vi "TablePicture.vi"(4 "RowIndex":i32, 5 "Font In":refnum<class "Font.lvclass">, 6 "Row Configuration":T1={"Cell Defaults"={"Background Color"=16777215, "Horizontal Align"=3, "Vertical Align"=1, "Minimum Height"=0.0, "Fixed Height"=0.0, "Padding"={"Left"=2.0, "Top"=2.0, "Right"=2.0, "Bottom"=3.0}}, "Row Borders"={"Left"={"Enabled"=TRUE, "Width"=0.5, "Color"=0}, "Top"={"Enabled"=TRUE, "Width"=0.75, "Color"=0}, "Right"={"Enabled"=TRUE, "Width"=0.5, "Color"=0}, "Bottom"={"Enabled"=TRUE, "Width"=0.75, "Color"=0}, "Middle Vertical"={"Enabled"=TRUE, "Width"=0.5, "Color"=0}}} {"Cell Defaults"."Vertical Align" items=["Bottom", "Middle", "Top"]; "Cell Defaults"."Horizontal Align" items=["Center", "Justified", "JustifiedAll", "Left", "Right"]}, 7 "TablePictures empty?":bool, 8 "Fehler (Eingang, kein Fehler)":errorcluster, 9 "Table in":string[](array[string]), 10 "TablePictures in":T4={"Ctl Refnum In"=[], "RowOrColumn"=enum."Row", "IndexToInsert"=0, "Image Scale (%)"=[], "Autoscale? (T)"=[], "Horizontal Align"=3} {"Horizontal Align" items=["Center", "Justified", "JustifiedAll", "Left", "Right"]}, 11 "Table Builder (Eingang)":refnum<class "Table Builder.lvclass">) -> (0 "Fehler (Ausgang)":errorcluster, 2 "Row Formatting out":refnum<class "Formatting.lvclass">[](array[class]), 3 "Table Builder (Ausgang)":refnum<class "Table Builder.lvclass">)   [LabVIEW 2020, in "PDF Interface.lvlib" / "PDF Interface Helper.lvlib"]
uses:
  PDF Interface Helper.lvlib
  <vilib>/Simplicity AI/SAI_PDF_API/Classes/Table Formatting/Formatting.lvclass
  <vilib>/Simplicity AI/SAI_PDF_API/Classes/Table Builder/Table Builder.lvclass
  PDFTablePictures.ctl
  <vilib>/Simplicity AI/SAI_PDF_API/Classes/Table Builder/Controls/SAI_PDF_Row Configuration.ctl
  <vilib>/Simplicity AI/SAI_PDF_API/Classes/Table Builder/Controls/SAI_PDF_Default Cell Format.ctl
  <vilib>/Simplicity AI/SAI_PDF_API/Classes/Table Builder/Controls/SAI_PDF_BorderLine.ctl
  <vilib>/Simplicity AI/SAI_PDF_API/Classes/Font/Font.lvclass
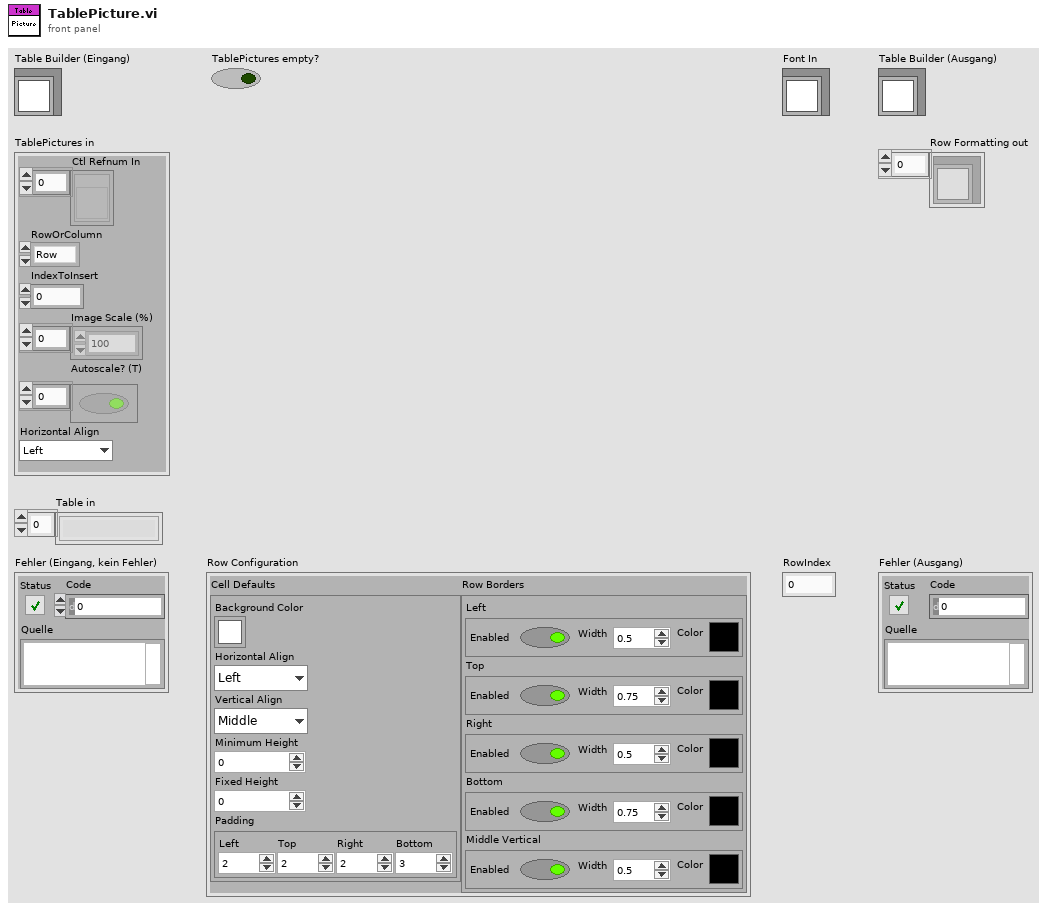
[diagram p1: front panel]
types:
  T1 = typedef "SAI_PDF_Toolkit.lvlib/Table Builder.lvclass/SAI_PDF_Row Configuration.ctl" = cluster{"Cell Defaults":T2, "Row Borders":cluster{"Left":T3, "Top":T3, "Right":T3, "Bottom":T3, "Middle Vertical":T3}}
  T2 = typedef "SAI_PDF_Toolkit.lvlib/Table Builder.lvclass/SAI_PDF_Default Cell Format.ctl" = cluster{"Background Color":u32, "Horizontal Align":i32, "Vertical Align":i32, "Minimum Height":sgl, "Fixed Height":sgl, "Padding":cluster{"Left":sgl, "Top":sgl, "Right":sgl, "Bottom":sgl}}
  T3 = typedef "SAI_PDF_Toolkit.lvlib/Table Builder.lvclass/SAI_PDF_BorderLine.ctl" = cluster{"Enabled":bool, "Width":sgl, "Color":u32}
  T4 = typedef "PDF Interface.lvlib/PDF Interface Helper.lvlib/PDFTablePictures.ctl" = cluster{"Ctl Refnum In":refnum<vi>[], "RowOrColumn":enum16{"Row", "Column"}, "IndexToInsert":u16, "Image Scale (%)":sgl[], "Autoscale? (T)":bool[], "Horizontal Align":i32}
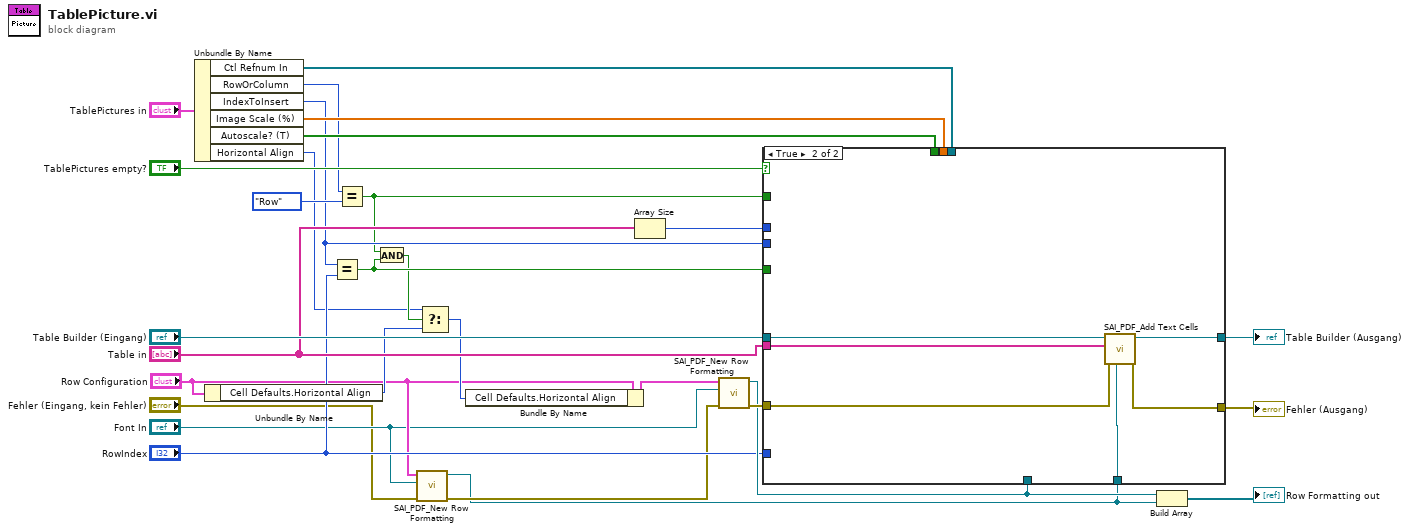
[diagram p0: block diagram]
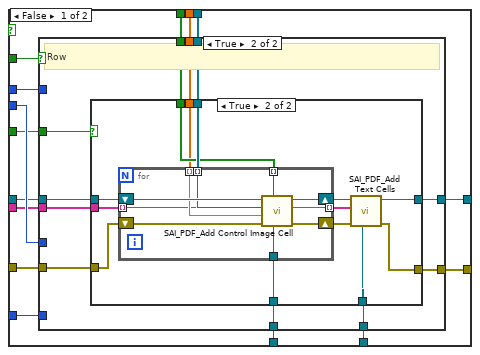
[diagram p2: hidden frame]
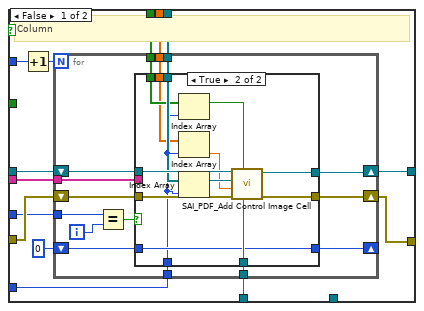
[diagram p3: hidden frame]
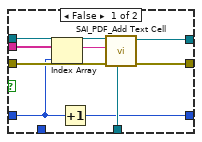
[diagram p4: hidden frame]
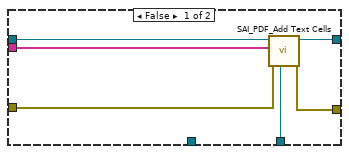
[diagram p5: hidden frame]
diagram:
  n1 = Unbundle By Name("TablePictures in") -> ("Ctl Refnum In"=w24:refnum<vi>[], "RowOrColumn"=w20:enum16{"Row", "Column"}, "IndexToInsert"=w14:u16, "Image Scale (%)"=w23:sgl[], "Autoscale? (T)"=w22:bool[], "Horizontal Align"=w9:i32)
  n2 = Unbundle By Name("Row Configuration") -> ("Cell Defaults.Horizontal Align"=w8:i32)
  n3 = Equal?(x=w14, y="RowIndex") -> (x = y?=w11:bool)
  n4 = Equal?(x=w20, y=enum16{"Row", "Column"}."Row") -> (x = y?=w12:bool)
  n5 = And(x=w12, y=w11) -> (x .and. y?=w10:bool)
  n6 = call <vilib>:"SAI_PDF_New Row Formatting.vi"("error in"="Fehler (Eingang, kein Fehler)", "Font In"="Font In", "Row Configuration"="Row Configuration") -> ("error out"=w3:errorcluster, "Row Formatting"=w1:refnum<class "Formatting.lvclass">)  [unwired: 7 out]
  n7 = Select(t=w9, s=w10, f=w8) -> (s? t:f=w7:i32)
  n8 = Bundle By Name(cluster="Row Configuration", "Cell Defaults.Horizontal Align"=w7) -> (w13:T1)
  n9 = Array Size(array="Table in") -> (size(s)=w18:i32)
  n10 = call <vilib>:"SAI_PDF_New Row Formatting.vi"("error in"=w3, "Font In"="Font In", "Row Configuration"=w13) -> ("error out"=w17:errorcluster, "Row Formatting"=w16:refnum<class "Formatting.lvclass">)  [unwired: 7 out]
  n11 = case shown="True" "TablePictures empty?" {
    tunnel: "Table Builder (Eingang)" -> [w41 w140]
    tunnel: "Table in" -> [w35 w139]
    tunnel: [w39 w138] -> w27
    tunnel: [w37 w137] -> w28
    tunnel: w17 -> [w38 w136]
    tunnel: w1 -> [w36 w135]
    tunnel: w12 -> [w44 _]
    tunnel: "RowIndex" -> [w43 _]
    tunnel: w14 -> [w42 _]
    tunnel: w16 -> [w40 _]
    tunnel: w24 -> [w34 _]
    tunnel: w23 -> [w33 _]
    tunnel: w22 -> [w32 _]
    tunnel: w18 -> [w31 _]
    tunnel: w11 -> [w30 _]
    frame False {
      n12 = case shown="True" w44 {
        tunnel: w43 -> [w50 _]
        tunnel: w42 -> [w52 _]
        tunnel: w41 -> [w57 w106]
        tunnel: w40 -> [w58 w105]
        tunnel: [w56 w104] -> w39
        tunnel: w38 -> [w54 w103]
        tunnel: [w53 w102] -> w37
        tunnel: w36 -> [_ w101]
        tunnel: w35 -> [w55 w100]
        tunnel: w34 -> [w51 w99]
        tunnel: w33 -> [w47 w98]
        tunnel: w32 -> [w48 w97]
        tunnel: w31 -> [w46 _]
        tunnel: w30 -> [_ w96]
        frame False {
          # "Column"
          n13 = Increment(x=w46) -> (x+1=w45:i32)
          n14 = for {
            N: w45 -> [_]
            tunnel: w58 -> [w73]
            shift-right: [w68] -> w56
            shift-left: w57 -> [w72]
            tunnel: w55 -> [w71]
            shift-right: [w69] -> w53
            shift-left: w54 -> [w70]
            tunnel: w52 -> [w66]
            tunnel: w51 -> [w65]
            tunnel: w50 -> [w64]
            shift-right: [w62] -> _
            shift-left: 0 -> [w61]
            tunnel: w48 -> [w60]
            tunnel: w47 -> [w59]
            i -> [w63]
            n15 = Equal?(x=w66, y=w63) -> (x = y?=w67:bool)
            n16 = case shown="True" w67 {
              tunnel: w73 -> [w82 w91]
              tunnel: w72 -> [w81 w95]
              tunnel: w71 -> [w80 _]
              tunnel: w70 -> [w79 w93]
              tunnel: [w78 w92] -> w69
              tunnel: [w77 w94] -> w68
              tunnel: w65 -> [_ w90]
              tunnel: w64 -> [_ w83]
              tunnel: w61 -> [w75 w88]
              tunnel: [w74 w88] -> w62
              tunnel: w60 -> [_ w87]
              tunnel: w59 -> [_ w85]
              frame False {
                n17 = Index Array(array=w80, index=w75) -> (element=w76:string)
                n18 = Increment(x=w75) -> (x+1=w74:i32)
                n19 = call <vilib>:"SAI_PDF_Add Text Cell.vi"("Formatting In"=w82, "error in"=w79, "Text"=w76, "Table Builder In"=w81) -> ("error out"=w78:errorcluster, "Table Builder Out"=w77:refnum<class "Table Builder.lvclass">)  [unwired: 6 in]
              }
              frame True {
                n20 = Index Array(array=w87, index=w83) -> (element=w86:bool)
                n21 = Index Array(array=w85, index=w83) -> (element=w84:sgl)
                n22 = Index Array(array=w90, index=w83) -> (element=w89:refnum<vi>)
                n23 = call <vilib>:"SAI_PDF_Add Control Image Cell.vi"("Formatting In"=w91, "Autoscale? (T)"=w86, "error in"=w93, "Image Scale (%)"=w84, "Ctl Refnum In"=w89, "Table Builder In"=w95) -> ("error out"=w92:errorcluster, "Table Builder Out"=w94:refnum<class "Table Builder.lvclass">)  [unwired: 4 in]
              }
            }
          }
        }
        frame True {
          # "Row"
          n24 = case shown="True" w96 {
            tunnel: w106 -> [w112 w125]
            tunnel: w105 -> [_ w124]
            tunnel: [w111 w122] -> w104
            tunnel: w103 -> [w109 w121]
            tunnel: [w110 w119] -> w102
            tunnel: w101 -> [w107 w118]
            tunnel: w100 -> [w108 w114]
            tunnel: w99 -> [_ w117]
            tunnel: w98 -> [_ w115]
            tunnel: w97 -> [_ w116]
            frame False {
              n25 = call <vilib>:"SAI_PDF_Add Text Cells.vi"("Formatting In"=w107, "error in"=w109, "Cell Text"=w108, "Table Builder In"=w112) -> ("error out"=w110:errorcluster, "Table Builder Out"=w111:refnum<class "Table Builder.lvclass">)  [unwired: 6 out]
            }
            frame True {
              n26 = for {
                tunnel: w124 -> [w133]
                shift-right: [w132] -> w123
                shift-left: w125 -> [w134]
                shift-right: [w130] -> w120
                shift-left: w121 -> [w131]
                tunnel: w117 -> [w129] mode=indexing
                tunnel: w116 -> [w128] mode=indexing
                tunnel: w115 -> [w127] mode=indexing
                tunnel: w114 -> [w126] mode=indexing
                tunnel: [w126] -> w113 mode=indexing
                n27 = call <vilib>:"SAI_PDF_Add Control Image Cell.vi"("Formatting In"=w133, "Autoscale? (T)"=w128, "error in"=w131, "Image Scale (%)"=w127, "Ctl Refnum In"=w129, "Table Builder In"=w134) -> ("error out"=w130:errorcluster, "Table Builder Out"=w132:refnum<class "Table Builder.lvclass">)  [unwired: 4 in]
              }
              n28 = call <vilib>:"SAI_PDF_Add Text Cells.vi"("Formatting In"=w118, "error in"=w120, "Cell Text"=w113, "Table Builder In"=w123) -> ("error out"=w119:errorcluster, "Table Builder Out"=w122:refnum<class "Table Builder.lvclass">)  [unwired: 6 out]
            }
          }
        }
      }
    }
    frame True {
      n29 = call <vilib>:"SAI_PDF_Add Text Cells.vi"("Formatting In"=w135, "error in"=w136, "Cell Text"=w139, "Table Builder In"=w140) -> ("error out"=w137:errorcluster, "Table Builder Out"=w138:refnum<class "Table Builder.lvclass">)  [unwired: 6 out]
    }
  }
  "Fehler (Ausgang)" <- w28
  "Table Builder (Ausgang)" <- w27
  n30 = Build Array(w16, w1) -> (→"Row Formatting out":refnum<class "Formatting.lvclass">[])
